vi "Config-Chan-VMUs.vi"(0 "VISA resource name":refnum<visa-resource-name>, 5 "VMU1 V name \n(max 6 chars)":string, 7 "VMU2 V name \n(max 6 chars)":string, 9 "VMU1/VMU2 mode (both disabled:0)":u16(ring) items=["VMU1 disabled, VMU2 disabled", "VMU1 V mode, VMU2 disabled", "VMU1 disabled, VMU2 V mode", "VMU1 V mode, VMU2 V mode", "differential voltage measurement"], 11 "error in (no error)":errorcluster) -> (4 "VISA resource name out":refnum<visa-resource-name>, 15 "error out":errorcluster)   [LabVIEW 2016, in "Agilent 415X Series.lvlib"]
doc: "This VI configures both VMUs of the HP415xA. \n\nThis VI corresponds to the Channel Definition Page of the instrument."
uses:
  Agilent 415X Series.lvlib
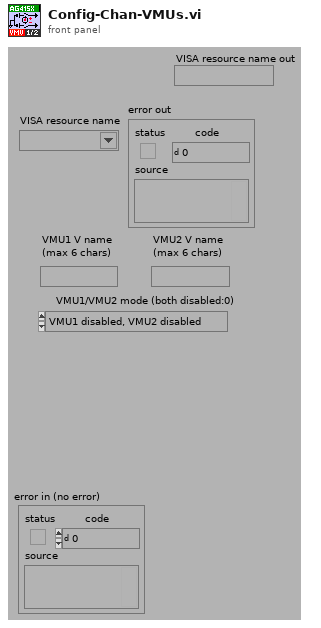
[diagram p1: front panel]
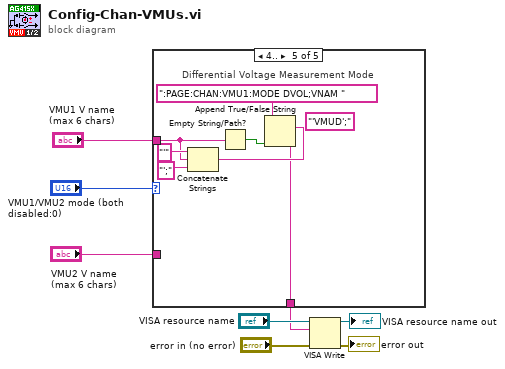
[diagram p0: block diagram]
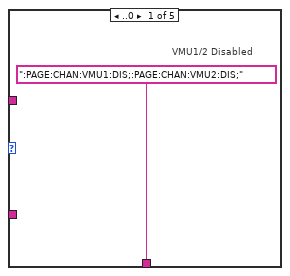
[diagram p2: hidden frame]
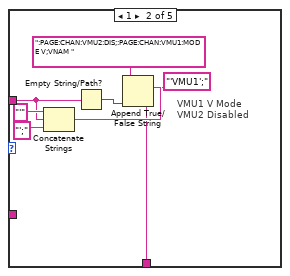
[diagram p3: hidden frame]
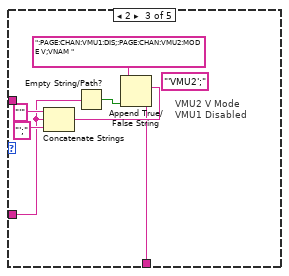
[diagram p4: hidden frame]
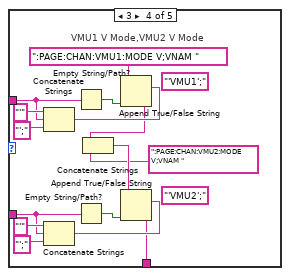
[diagram p5: hidden frame]
diagram:
  n1 = case shown="4.." "VMU1/VMU2 mode (both disabled:0)" {
    tunnel: "VMU1 V name \n(max 6 chars)" -> [_ w15 _ w40 w48]
    tunnel: [":PAGE:CHAN:VMU1:DIS;:PAGE:CHAN:VMU2:DIS;" w10 w19 w29 w43] -> w2
    tunnel: "VMU2 V name \n(max 6 chars)" -> [_ _ w18 w31 _]
    frame ..0 {
      # "VMU1/2 Disabled"
    }
    frame 1 {
      # "VMU1 V Mode\nVMU2 Disabled"
      n2 = Concatenate Strings("'", w15, "';") -> (w14:string)
      n3 = Empty String/Path?(string/path=w15) -> (empty?=w17:bool)
      n4 = Append True/False String(1:w17, 2:w14, 3:"'VMU1';", 4:":PAGE:CHAN:VMU2:DIS;:PAGE:CHAN:VMU1:MODE V;VNAM ") -> (0:w10:string)
    }
    frame 2 {
      # "VMU2 V Mode\nVMU1 Disabled"
      n5 = Concatenate Strings("'", w18, "';") -> (w23:string)
      n6 = Empty String/Path?(string/path=w18) -> (empty?=w25:bool)
      n7 = Append True/False String(1:w25, 2:w23, 3:"'VMU2';", 4:":PAGE:CHAN:VMU1:DIS;:PAGE:CHAN:VMU2:MODE V;VNAM ") -> (0:w19:string)
    }
    frame 3 {
      # "VMU1 V Mode,VMU2 V Mode"
      n8 = Concatenate Strings("'", w40, "';") -> (w39:string)
      n9 = Concatenate Strings("'", w31, "';") -> (w34:string)
      n10 = Empty String/Path?(string/path=w40) -> (empty?=w42:bool)
      n11 = Empty String/Path?(string/path=w31) -> (empty?=w32:bool)
      n12 = Append True/False String(1:w42, 2:w39, 3:"'VMU1';", 4:":PAGE:CHAN:VMU1:MODE V;VNAM ") -> (0:w27:string)
      n13 = Concatenate Strings(w27, ":PAGE:CHAN:VMU2:MODE V;VNAM ") -> (w28:string)
      n14 = Append True/False String(1:w32, 2:w34, 3:"'VMU2';", 4:w28) -> (0:w29:string)
    }
    frame 4.. {
      # "Differential Voltage Measurement Mode"
      n15 = Concatenate Strings("'", w48, "';") -> (w47:string)
      n16 = Empty String/Path?(string/path=w48) -> (empty?=w50:bool)
      n17 = Append True/False String(1:w50, 2:w47, 3:"'VMUD';", 4:":PAGE:CHAN:VMU1:MODE DVOL;VNAM ") -> (0:w43:string)
    }
  }
  n18 = VISA Write(VISA resource name="VISA resource name", write buffer=w2, error in (no error)="error in (no error)") -> (VISA resource name out=→"VISA resource name out":refnum<visa-resource-name>, error out=→"error out":errorcluster)  [unwired: 1 out]
